vi "Command Stopped.vi"(8 "error in (no error)":errorcluster, 9 "Command Name (Instance)":string, 10 "final error code":i32, 11 "Running Command in":refnum<class "Running Command.lvclass">) -> (0 "error out":errorcluster, 3 "Running Command out":refnum<class "Running Command.lvclass">)   [LabVIEW 2014, in "Robot Actor Framework.lvlib" / "Command Processor Actor.lvlib" / "Running Command.lvclass"]
uses:
  Running Command.lvclass
  <vilib>/ActorFramework/Message Enqueuer/Message Priority.ctl
  <vilib>/ActorFramework/Actor/Actor.lvclass/Actor.ctl
  <vilib>/ActorFramework/Message Enqueuer/Message Enqueuer.lvclass/Message Enqueuer.ctl
  <vilib>/ActorFramework/Message Enqueuer/Init from Existing Queue.vi
  <vilib>/ActorFramework/Message Enqueuer/Enqueue.vi
  <vilib>/ActorFramework/Message Priority Queue/Priority Enqueue.vi
  Command Processor Actor Class/Command Processor Actor.lvclass
  <vilib>/ActorFramework/Message Enqueuer/Message Enqueuer.lvclass
  Command Processor Actor Messages/Go To No Command Msg/Go To No Command Msg.lvclass
  <vilib>/ActorFramework/Actor/Actor.lvclass
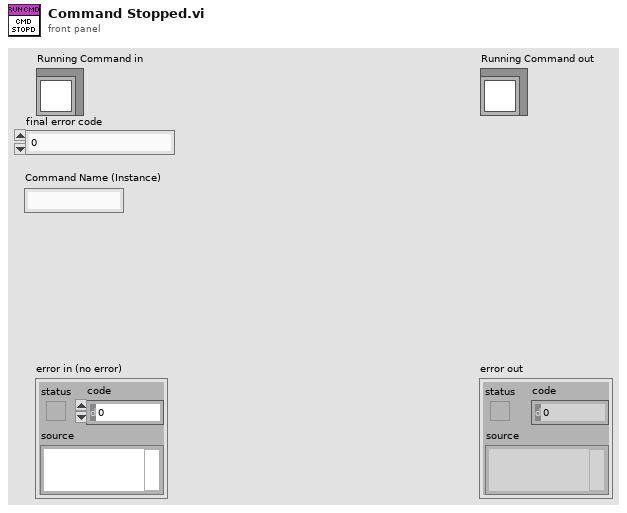
[diagram p1: front panel]
types:
  T1 = typedef "Actor Framework.lvlib/Message Enqueuer.lvclass/Message Priority.ctl" = enum16{"Low", "Normal", "High"}
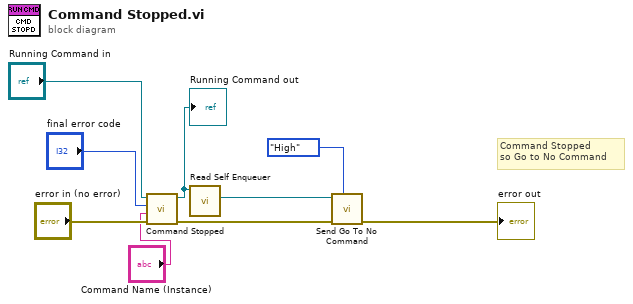
[diagram p0: block diagram]
diagram:
  # "Command Stopped\nso Go to No Command"
  n1 = call-parent "Command Stopped.vi"("error in (no error)"="error in (no error)", "Command Name (Instance)"="Command Name (Instance)", "final error code"="final error code", "Command Processor Actor in"="Running Command in") -> ("error out"=w3:errorcluster, "Command Processor Actor out"=w4:refnum<class "Running Command.lvclass">)  [unwired: 6 in]
  "Running Command out" <- w4
  n2 = call <vilib>:"Read Self Enqueuer.vi"("Actor"=w4) -> ("Self Enqueuer"=w8:refnum<class "Message Enqueuer.lvclass">)  [unwired: 10 in]
  n3 = call "Send Go To No Command.vi"("Message Priority (Normal)"=Message_Priority."High", "error in (no error)"=w3, "Message Enqueuer"=w8) -> ("error out"=→"error out":errorcluster)  [unwired: 7 in, 1 out]
